vi "Offset Inline Buffers.vi"(8 "error in (no error)":errorcluster, 10 "Command Parameters":T1, 11 "Dispatcher in":refnum<class "Dispatcher.lvclass">) -> (0 "error out":errorcluster, 3 "Dispatcher out":refnum<class "Dispatcher.lvclass">)   [LabVIEW 2017, in "DSF Core.lvlib" / "Dispatcher.lvclass"]
uses:
  Dispatcher.lvclass
  <vilib>/NI/Memory Manager/Classes/Pointer/Memory.Pointer.lvclass
  Plugin/Plugin.lvclass
  Interfaces/Dispatcher/Command Parameters.ctl
  Interfaces/Dispatcher/Dispatcher Interface.lvclass
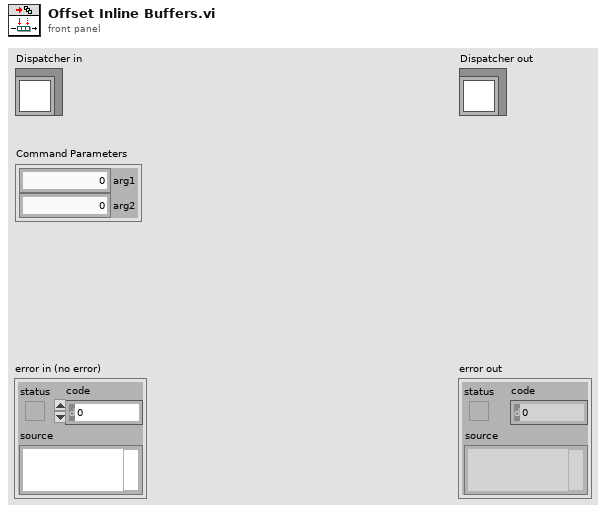
[diagram p1: front panel]
types:
  T1 = typedef "DSF Core.lvlib/Dispatcher Interface.lvclass/Command Parameters.ctl" = cluster{"arg1":u64, "arg2":u64}
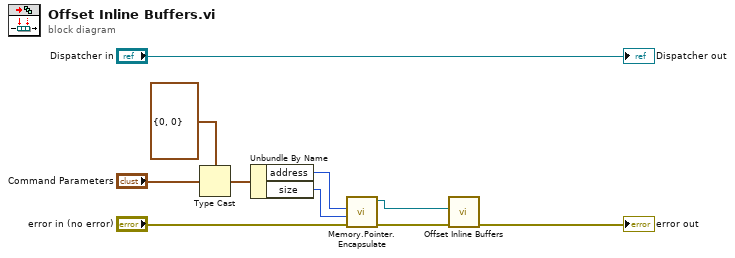
[diagram p0: block diagram]
diagram:
  n1 = Type Cast(type=cluster{"address":u64, "size":u64} {"address"=0, "size"=0}, x="Command Parameters") -> (*(type *) &x=w7:cluster{"address":u64, "size":u64})
  n2 = Unbundle By Name(w7) -> ("address"=w4:u64, "size"=w5:u64)
  n3 = call <vilib>:"Memory.Pointer.Encapsulate.vi"("error in (no error)"="error in (no error)", "size"=w5, "address"=w4) -> ("error out"=w3:errorcluster, "Pointer out"=w1:refnum<class "Memory.Pointer.lvclass">)  [unwired: 7 in]
  n4 = call "Offset Inline Buffers.vi"("error in (no error)"=w3, "Engine Pointer"=w1) -> ("error out"=→"error out":errorcluster)  [unwired: 8 in, 1 out]
  "Dispatcher out" <- "Dispatcher in"
